vi "Update Dir Value.vi"(9 "Value":i32, 10 "Map in":map{string, i32}(c390), 11 "Current dir":string) -> (3 "Map out":map{string, i32}(c390))   [LabVIEW 2021]
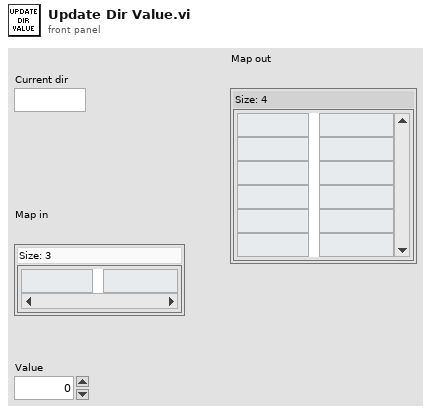
[diagram p1: front panel]
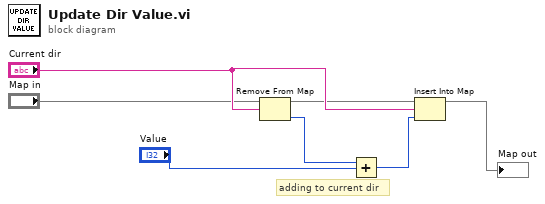
[diagram p0: block diagram]
diagram:
  # "adding to current dir"
  n1 = Remove From Map(10:"Current dir", 11:"Map in") -> (1:w6:i32, 3:w4:map{string, i32})  [unwired: 1 out]
  n2 = Add(x=w6, y="Value") -> (x+y=w2:i32)
  n3 = Insert Into Map(map in=w4, key="Current dir", value=w2) -> (map out=→"Map out":map{string, i32})  [unwired: 2 out]
